vi "电能清零.vi"(3 "串口号":refnum<visa-resource-name>) -> (1 "应答":string)   [LabVIEW 2014]
panel:
  in  "保留参数":u8
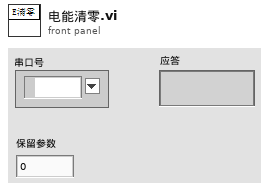
[diagram p1: front panel]
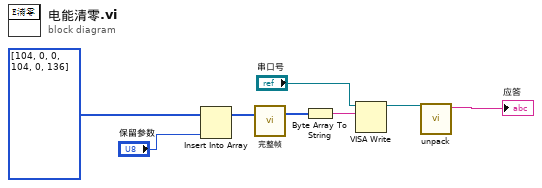
[diagram p0: block diagram]
diagram:
  n1 = Insert Into Array(array=u8[] [104, 0, 0, 104, 0, 136], new element="保留参数") -> (w2:u8[])  [unwired: 1 in]
  n2 = call "完整帧.vi"("不完整帧"=w2) -> ("完整帧"=w3:u8[])  [unwired: 2 in]
  n3 = Byte Array To String(unsigned byte array=w3) -> (string=w4:string)
  n4 = VISA Write(VISA resource name="串口号", write buffer=w4) -> (VISA resource name out=w6:refnum<visa-resource-name>)  [unwired: 1 in, 2 out]
  n5 = call "unpack.vi"("串口号输入"=w6) -> ("应答"=→"应答":string)  [unwired: 5 in, 1 out]
